vi "ReadBaseActor.vi"(7 "Actor in":refnum<class "Actor.lvclass">) -> (3 "BaseActor":T1)   [LabVIEW 2020, in "jettl.lvlib" / "Actor.lvclass"]
uses:
  Actor.lvclass
  Message/Message.lvclass
  ActorLifetime.ctl
  jettl.lvlib
  MessageSet.ctl
  Messages.ctl
  Message.ctl
  ActorType.ctl
  Actor.ctl
  ActorMap.ctl
  BaseActor.ctl
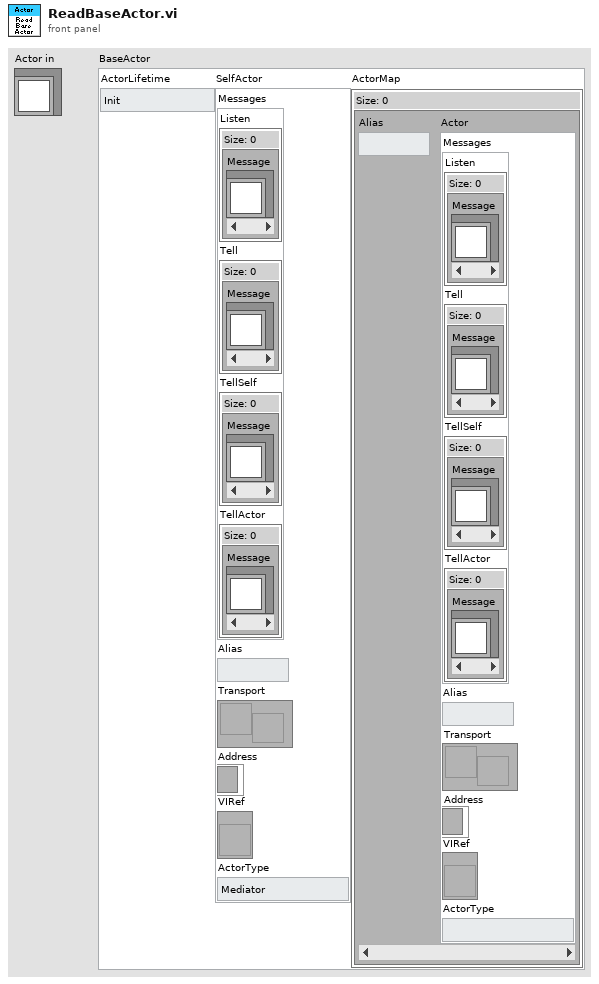
[diagram p1: front panel]
types:
  T1 = typedef "jettl.lvlib/BaseActor.ctl" = cluster{"ActorLifetime":T2, "SelfActor":T3, "ActorMap":T7}
  T2 = typedef "jettl.lvlib/ActorLifetime.ctl" = enum16{"Init", "Spawn", "Setup", "Teardown Before Running", "Running", "Stop Called", "Stopping With Children", "Stopping Without Children", "Teardown After Running", "Stopped"}
  T3 = typedef "jettl.lvlib/Actor.ctl" = cluster{"Messages":T4, "Alias":string, "Transport":refnum<user-event>, "Address":refnum<event-registration>, "VIRef":refnum<vi>, "ActorType":T6}
  T4 = typedef "jettl.lvlib/Messages.ctl" = cluster{"Listen":T5, "Tell":T5, "TellSelf":T5, "TellActor":T5}
  T5 = typedef "jettl.lvlib/MessageSet.ctl" = set{refnum<class "Message.lvclass">}
  T6 = typedef "jettl.lvlib/ActorType.ctl" = enum16{"Mediator", "Component"}
  T7 = typedef "jettl.lvlib/ActorMap.ctl" = map{string, T3}
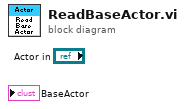
[diagram p0: block diagram]
diagram:
